vi "XYStage.GetPosition.vi"(8 "error in (no error)":errorcluster, 11 "XYStage in":refnum<class "XYStage.lvclass">) -> (0 "error out":errorcluster, 2 "Coordinates":T1, 3 "XYStage out":refnum<class "XYStage.lvclass">)   [LabVIEW 2019, in "XYStage.lvclass"]
uses:
  XYStage.lvclass
  Typedefs/Coordinates--Cluster.ctl
  Typedefs/Coordinates.Units--Cluster.ctl
  Typedefs/Coordinates.Counts--Cluster.ctl
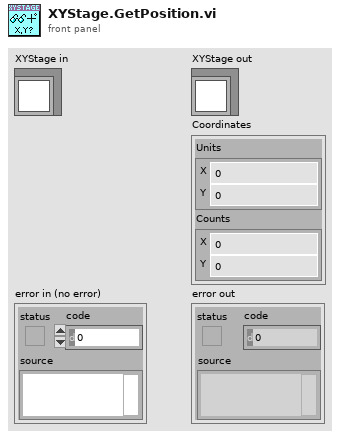
[diagram p1: front panel]
types:
  T1 = typedef "XYStage.lvclass/Coordinates--Cluster.ctl" = cluster{"Units":T2, "Counts":T3}
  T2 = typedef "XYStage.lvclass/Coordinates.Units--Cluster.ctl" = cluster{"X":dbl, "Y":dbl}
  T3 = typedef "XYStage.lvclass/Coordinates.Counts--Cluster.ctl" = cluster{"X":i32, "Y":i32}
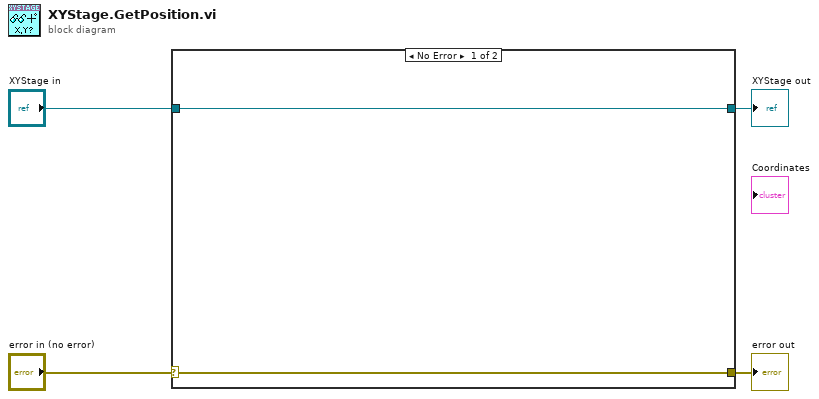
[diagram p0: block diagram]
diagram:
  n1 = case shown="No Error" "error in (no error)" {
    selector: "error in (no error)" -> [w5 w8]
    tunnel: [w5 w8] -> w3
    tunnel: [w6 w7] -> w1
    tunnel: "XYStage in" -> [w6 w7]
    frame No Error {
    }
    frame Error {
    }
  }
  "error out" <- w3
  "XYStage out" <- w1
